vi "NanotecSMCPDDriver.set address.vi"(0 "VISA resource name":refnum<visa-resource-name>, 1 "contollerID":i32=-1, 3 "address":i32, 5 "error in (no error)":errorcluster) -> (14 "VISA resource name out":refnum<visa-resource-name>, 15 "contollerID out":i32=-1, 19 "error out":errorcluster)   [LabVIEW 2014, in "NanotecSMCPDDriver.lvlib"]
doc: "Sets the address of the controller. Please make sure, that the addresses of all controllers on the serial bus are unique. \n\nComment: It might be useful, to use the \"getAddress\" VI in order to obtain an unknown address of a controller."
uses:
  NanotecSMCPDDriver.lvlib
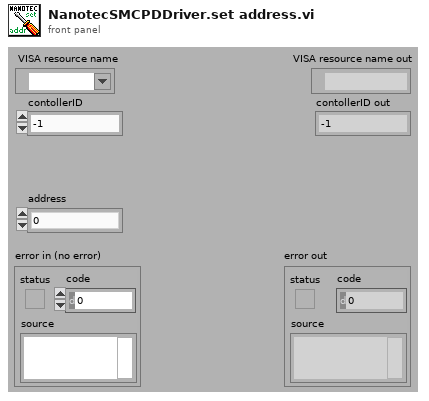
[diagram p1: front panel]
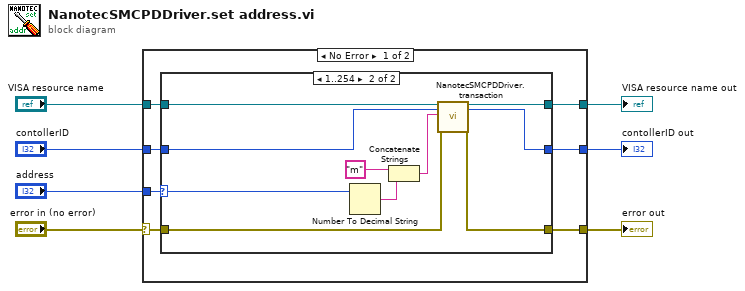
[diagram p0: block diagram]
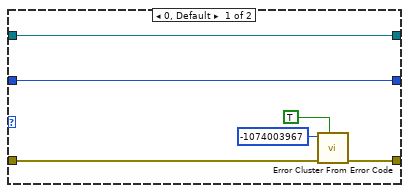
[diagram p2: hidden frame]
diagram:
  n1 = case shown="No Error" "error in (no error)" {
    selector: "error in (no error)" -> [w9 w31]
    tunnel: [w11 w33] -> w7
    tunnel: [w10 w31] -> w6
    tunnel: "VISA resource name" -> [w14 w33]
    tunnel: "contollerID" -> [w13 w32]
    tunnel: [w12 w32] -> w3
    tunnel: "address" -> [w8 _]
    frame No Error {
      n2 = case shown="1..254" w8 {
        selector: w8 -> [_ w21]
        tunnel: w14 -> [w20 w30]
        tunnel: w13 -> [w15 w29]
        tunnel: [w15 w28] -> w12
        tunnel: [w20 w27] -> w11
        tunnel: [w19 w26] -> w10
        tunnel: w9 -> [w18 w25]
        frame 0, Default {
          n3 = call <vilib>:"Error Cluster From Error Code.vi"("show call chain? (False)"=TRUE, "error in (no error)"=w18, "error code (0)"=-1074003967) -> ("error out"=w19:errorcluster)  [unwired: 6 in]
        }
        frame 1..254 {
          n4 = Number To Decimal String(number=w21) -> (decimal integer string=w24:string)  [unwired: 1 in]
          n5 = Concatenate Strings("m" ("commandString"), w24) -> (w22:string)
          n6 = call "NanotecSMCPDDriver.transaction.vi"("VISAresource"=w30, "contollerID"=w29, "commandString"=w22, "error in (no error)"=w25) -> ("VISAresource out"=w27:refnum<visa-resource-name>, "contollerID out"=w28:i32, "error out"=w26:errorcluster)  [unwired: 10 in, 3 out]
        }
      }
    }
    frame Error {
    }
  }
  "VISA resource name out" <- w7
  "error out" <- w6
  "contollerID out" <- w3
